vi "LuaVIEW Cleanup Public Registry.vi"() -> (15 "error out":errorcluster)   [LabVIEW 2013]
doc: "Requests a cleanup of the public LuaVIEW function registry. This will cause the public function VIs as well as the registry daemon to be unloaded. Use of this VI is not necessary when the \"Unload Functions ASAP\" global is set. If the registry is not initialized, this function will return immediately. If the registry is still in use (there are running scripts that use public functions), this VI will fail. If the registry was initialized but no longer in use, this VI will return after unloading completes. Do not simultaneously register and cleanup."
uses:
  typedefs/t_LuaVIEW Daemon Exchange Methods.ctl
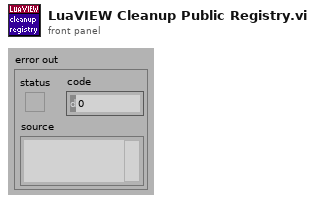
[diagram p1: front panel]
types:
  T1 = typedef "t_LuaVIEW Daemon Exchange Methods.ctl" = enum16{"inert", "send path", "send cleanup", "get sent", "reply", "get reply", "unset launched"}
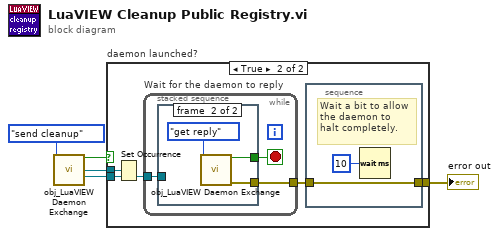
[diagram p0: block diagram]
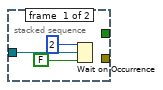
[diagram p3: hidden frame]
diagram:
  n1 = call "obj_LuaVIEW Daemon Exchange.vi"("method"=t_LuaVIEW_Daemon_Exchange_Methods."send cleanup") -> ("available?"=w2:bool, "send occurrence"=w4:refnum<k4>, "reply occurrence"=w3:refnum<k4>)  [unwired: 10 in, 2 out]
  n2 = case "daemon launched?" shown="True" w2 {
    tunnel: w4 -> [_ w9]
    tunnel: w3 -> [_ w8]
    tunnel: [_ w6] -> w1
    frame False {
    }
    frame True {
      n3 = Set Occurrence(w9) -> ()
      n4 = while "Wait for the daemon to reply" {
        tunnel: w8 -> [w14]
        tunnel: [w12] -> w7
        stop <- w13 stop-if-true
        n5 = stacked-sequence {
          tunnel: w14 -> [w17 _]
          tunnel: [_ w19] -> w13
          tunnel: [_ w18] -> w12
          frame #0 {
            n6 = Wait on Occurrence(1:FALSE ("ignore previous (T)"), 2:w17, 3:2 ("ms timeout (-1)")) -> ()  [unwired: 1 out]
          }
          frame #1 {
            n7 = call "obj_LuaVIEW Daemon Exchange.vi"("method"=t_LuaVIEW_Daemon_Exchange_Methods."get reply") -> ("available?"=w19:bool, "error reply out"=w18:errorcluster)  [unwired: 10 in, 3 out]
          }
        }
      }
      n8 = stacked-sequence {
        tunnel: [w11] -> w6
        tunnel: w7 -> [w11]
        frame #0 {
          # "Wait a bit to allow\nthe daemon to\nhalt completely."
          n9 = Wait (ms)(milliseconds to wait=u32 10) -> ()  [unwired: 1 out]
        }
      }
    }
  }
  "error out" <- w1
